vi "Scope_5782_Dual_PID.vi"() -> ()   [LabVIEW 2013]
uses:
  <vilib>/userdefined/High Color/nirio_resource_hc.ctl
  FPGA/DataMode.ctl
  <vilib>/Analysis/4window.llb/windowTd.ctl
  Host/Scope/controls/power_spectrum_unit.ctl
  Host/Scope5782/Scope/controls/5782_trigger_type.ctl
  Host/Scope/controls/Data_calc_mode.ctl
  Host/Scope/controls/Data_display_mode.ctl
  Host/Scope/controls/Graph_references.ctl
  Host/Scope/controls/graph_controls.ctl
  Host/Scope/controls/Channel_select.ctl
  Host/Communication/response.ctl
  Host/Communication/driver_status.ctl
  Host/Communication/Driver/RemoteConnection/RemoteReferences.ctl
  Host/Communication/Driver/TcpServerDriver/TcpServerDriver.lvclass
  Host/Scope5782/Scope/controls/c_t_type.ctl
  Host/Scope/controls/ScopeMode.ctl
  FPGA/fpga_settings.ctl
  Host/Communication/global_stop.vi
  <vilib>/FPGAPlugInAG/PXIe-7975R/niLvFpga_Open_PXIe-7975R.vi
  <vilib>/rvi/interface/common/dynamic/niFpgaDynamicAddResources.vi
  <vilib>/rvi/interface/common/niFpgaWaitOnOcc.vi
  <vilib>/Utility/error.llb/Error Cluster From Error Code.vi
  <vilib>/rvi/errors/niLvFpgaAdjustHostInterfaceError.vi
  <vilib>/FPGAPlugInAG/Dynamic/niLvFpga_Close_Dynamic.vi
  <vilib>/rvi/interface/nirviOpenFPGA/nirviOpenFPGA.xnode
  FPGA Bitfiles/FPGAmain_5782_Dual_PID_1Hh0+AVfYHk.lvbitx
  <vilib>/rvi/interface/nirviReadWriteControl/nirviReadWriteControl.xnode
  Host/Scope5782/Config/FPGAref_5782.ctl
  <vilib>/rvi/FXPMathLib/FxpInterpret/XNode/nifxpmath_Interpret.xnode
  <vilib>/rvi/interface/nirviMethod/nirviMethod.xnode
  <vilib>/rvi/interface/nirviCloseFPGA/nirviCloseFPGA.xnode
  Host/Utilities/Ticker/Ticker.lvclass
  NiFpgaLv.dll
  <vilib>/rvi/interface/Simulation/niFpgaSimulationCallBeginRW.vi
  Host/Communication/Driver/RemoteConnection/RemoteConnection.lvclass
  <vilib>/FPGAPlugInAG/Dynamic/niLvFpga_WriteFifo_Dynamic.vi
  <vilib>/rvi/errors/niLvFpgaMergeErrorWithErrorCode.vi
  <vilib>/Analysis/NI_AALPro.lvlib
panel:
  in  "Output enabled":bool=TRUE
  in  "unwrap phase":bool
  in  "Kp AM":fxp<+/-,32,4> caption="Kp"
  in  "Kd/T AM":fxp<+/-,32,4> caption="Kd/T"
  in  "Ki*T AM":fxp<+/-,32,4> caption="Ki*T"
  in  "Feedback AM":bool caption="Feedback"
  in  "c(t) AM":bool
  in  "c(t) phase":bool
  in  "Kp":fxp<+/-,32,4>
  in  "Kd/T":fxp<+/-,32,4>
  in  "Ki*T":fxp<+/-,32,4>
  in  "Feedback":bool
  in  "b":fxp<+/-,16,2>
  in  "a":fxp<+/-,16,2>
  in  "Fequency [kHz]":dbl format="%#_8g"
  in  "#bins":i32=1 min=1 max=16
  in  "ch1 DC offset":dbl caption="DC offset\nChannel 1"
  in  "ch0 DC offset":dbl caption="DC offset\nChannel 0"
  in  "Output delay delta":dbl(slide) scale=0.0..6.0
  in  "Output delay":dbl(slide) scale=0.0..6.0
  in  "Chart length":i32=200000
  in  "Trigmode":enum32{"Triggered", "Continuous"}(radio)
  in  "Refence for phase":T1
  in  "Graph_refs":T2
  out "Lower chart":dbl[][](graph)
  out "Upper chart":dbl[][](graph)
  out "Lower graph":i16[][](graph)
  in  "Buffer":T4
  in  "Display":T5
  in  "Output mixer fequency [MHz]":dbl
  in  "Trigger":T6
  in  "Ch1 Q":bool
  in  "Ch1 I":bool
  in  "Ch0 Q":bool
  in  "Ch0 I":bool
  in  "Ch1":bool
  in  "Ch0":bool
  out "stop 2":bool
  in  "Zoom freq X":bool
  in  "Zoom freq Y":bool
  in  "Zoom time Y":bool
  in  "Zoom time X":bool
  in  "Unit":T7
  in  "Window":T8=1 items=["Rectangle"=0, "Hanning"=1, "Hamming"=2, "Blackman-Harris"=3, "Exact Blackman"=4, "Blackman"=5, "Flat Top"=6, "4 Term B-Harris "=7, "7 Term B-Harris"=8, "Low Sidelobe"=9, "Blackman Nuttall"=11, "Triangle"=30, "Bartlett-Hanning"=31, "Bohman"=32, "Parzen"=33, "Welch"=34, "Kaiser"=60, "Dolph-Chebyshev"=61, "Gaussian"=62]
  in  "Samples per 5782 record":i32
  in  "Phase offset (deg)":dbl
  in  "Fequency [MHz]":dbl format="%#_8g"
  in  "Mode":T9
  in  "Mixer freq [MHz]":dbl
  out "freqdata":cluster{"f0":dbl, "df":dbl, "magnitude":dbl[]}[](graph)
  out "Upper graph":i16[][](graph)
  in  "Rumode":bool
  in  "Singleshot":bool
  out "error IO":errorcluster
  in  "stop":bool
  in  "resource name":T10="RIO0"
  out "Clocking Option Configured?":bool
  out "Configured?":bool
  # "FPGA setup"
  # "V"
  # "V"
  # "Output delay"
  # "ns"
  # "Auto Zoom"
  # "Output delay delta"
  # "ps"
  # "Amplitude modulation"
  # "5782"
  # "Phase"
  # "Amplitude"
  # "Simulated data"
  # "FFT"
  # "Auto Zoom"
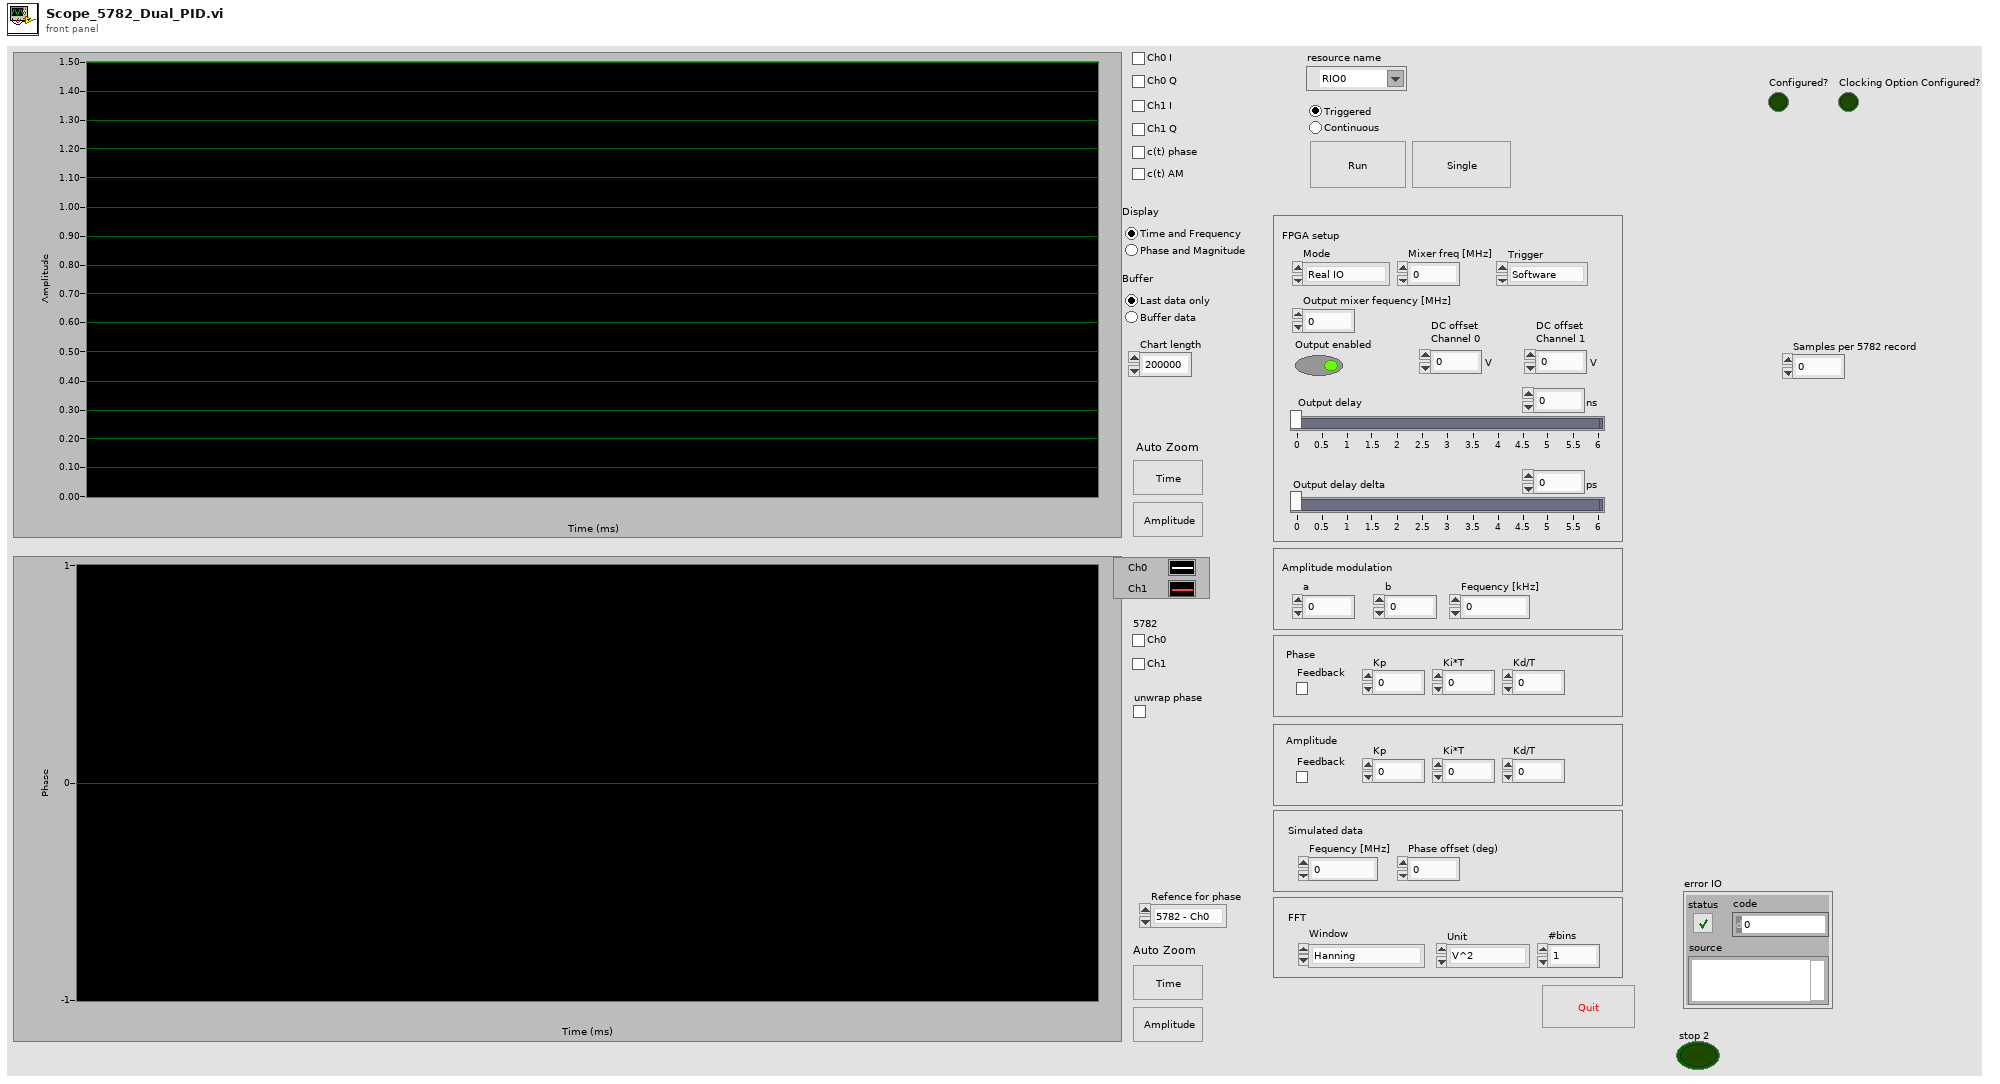
[diagram p1: front panel]
types:
  T1 = typedef "Channel_select.ctl" = enum16{"5782 - Ch0", "5782 - Ch1"}
  T2 = typedef "Graph_references.ctl" = cluster{"upper":T3, "lower":T3, "Freq graph":refnum<vi>}
  T3 = typedef "graph_controls.ctl" = cluster{"Graph":refnum<vi>, "Time btn":refnum<vi>, "Amplitude btn":refnum<vi>, "Chart":refnum<vi>}
  T4 = typedef "Data_display_mode.ctl" = enum32{"Last data only", "Buffer data"}
  T5 = typedef "Data_calc_mode.ctl" = enum32{"Time and Frequency", "Phase and Magnitude"}
  T6 = typedef "5782_trigger_type.ctl" = enum16{"Software", "Trigger input"}
  T7 = typedef "power_spectrum_unit.ctl" = enum16{"V^2", "V", "dBV"}
  T8 = typedef "NI_AALPro.lvlib/windowTd.ctl" = u32
  T9 = typedef "DataMode.ctl" = enum16{"Real IO", "Simulated"}
  T10 = typedef "nirio_resource_hc.ctl" = tag
  T11 = typedef "RemoteConnection.lvclass/RemoteReferences.ctl" = cluster{"a":refnum<vi>, "b":refnum<vi>, "fm":refnum<vi>, "Output delay":refnum<vi>, "Output delay delta":refnum<vi>}
  T12 = typedef "response.ctl" = cluster{"driver status":T13, "Sender":string, "Type":i32, "Variant":variant}
  T13 = typedef "driver_status.ctl" = enum16{"Normal", "Startup", "Connection lost", "Reconnected", "Timeout", "Idle", "Busy"}
  T14 = enum8{"Internal Clock PLL Off", "Internal Clock PLL On (REF IN)", "External Clock (CLK_IN)", "Internal Clock PLL On (IoModSyncClk)"}
  T15 = typedef "message_queue.ctl" = refnum<queue>
  T16 = typedef "FPGAref_5782.ctl" = refnum<k20>
  T17 = typedef "scope_params_5782.ctl" = cluster{"scope mode":T18, "ticker":refnum<class "Ticker.lvclass">, "samples per record":i32, "FPGA ref":T16, "data mode":T9, "5782 Trigger":T6, "Chart length":i32, "RemoteConnection":refnum<class "RemoteConnection.lvclass">, "last phase":dbl[]}
  T18 = typedef "ScopeMode.ctl" = enum16{"Stopped", "Single", "Running", "Continuous"}
  T19 = typedef "c_t_type.ctl" = enum16{"Phase", "AM", "Both"}
  T20 = typedef "fpga_settings.ctl" = enum16{"Feedback Enable", "New FIR coeffs", "FIR shift", "Enable filter", "Set Downsample", "Downsample", "CIC Gain", "Record length", "Trigger samples", "Quiet time", "a_am", "b_am", "Use fixed delay", "fixed sin_fi", "fixed cos_fi", "Ki*Tau", "Kp", "Kd_Tau", "Fi_start", "Fi_delta", "DC_offs 0", "DC_offs 1", "Ki*Tau am", "Kp am", "Kd_Tau am", "Feedback AM"}
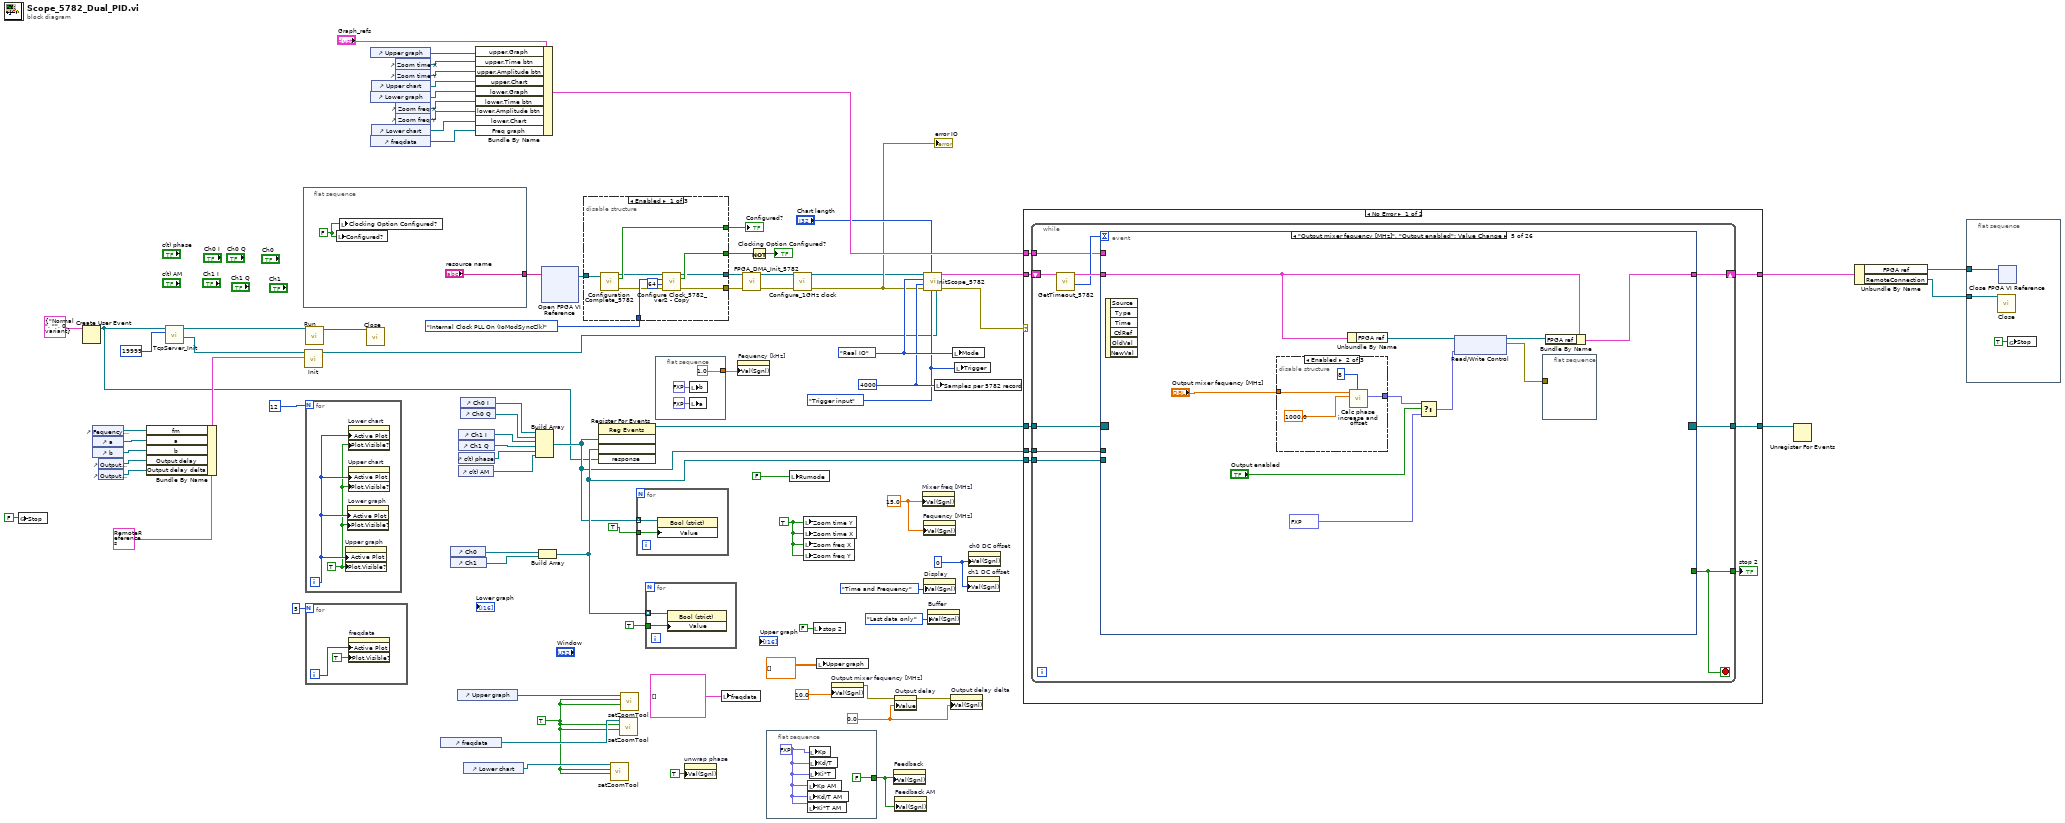
[diagram p0: block diagram]
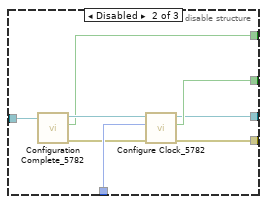
[diagram p2: hidden frame]
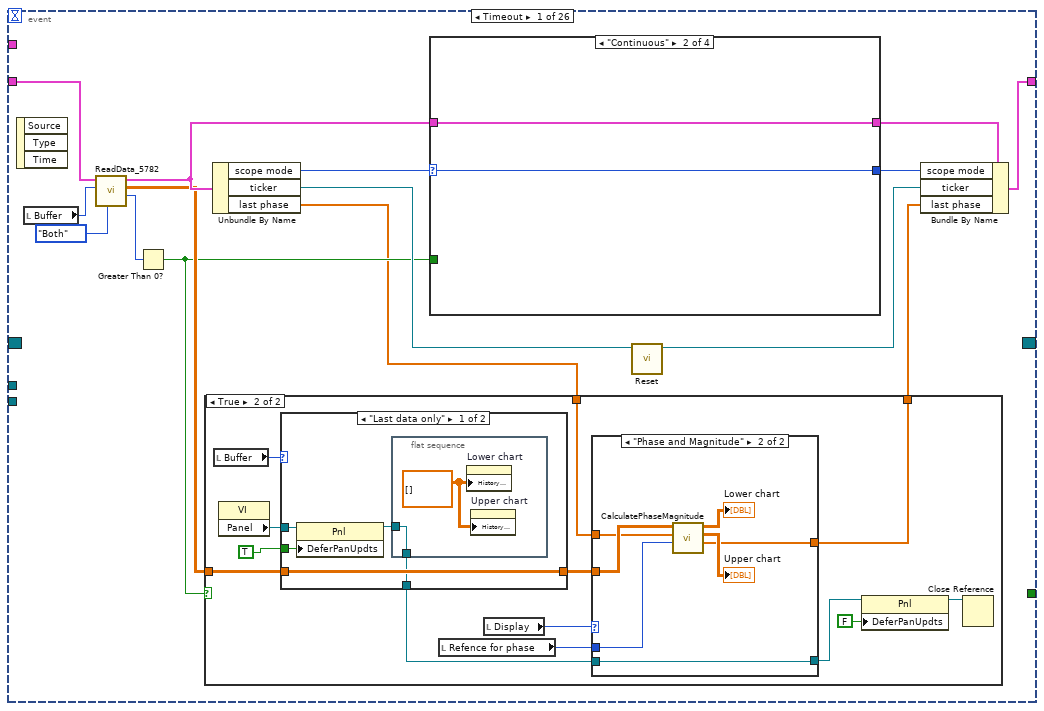
[diagram p4: hidden frame]
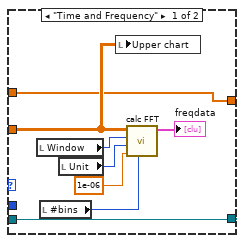
[diagram p7: hidden frame]
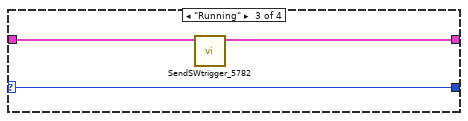
[diagram p9: hidden frame]
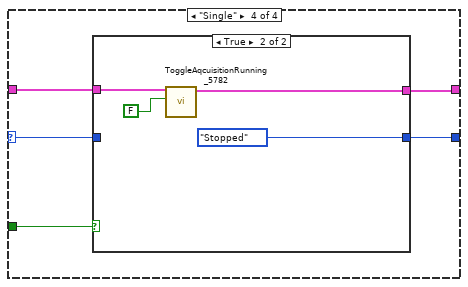
[diagram p10: hidden frame]
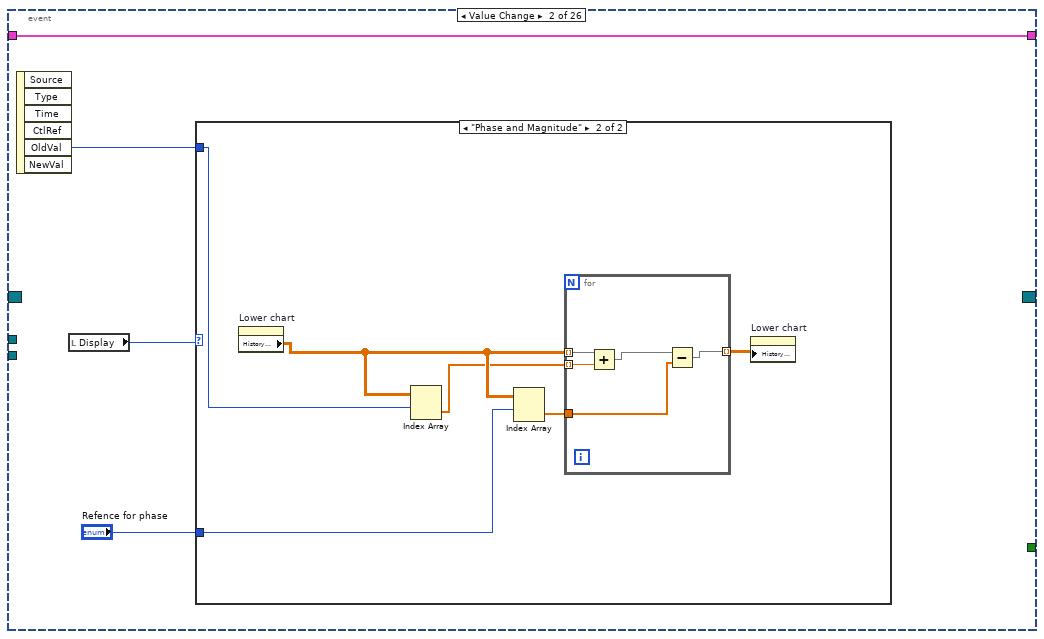
[diagram p12: hidden frame]
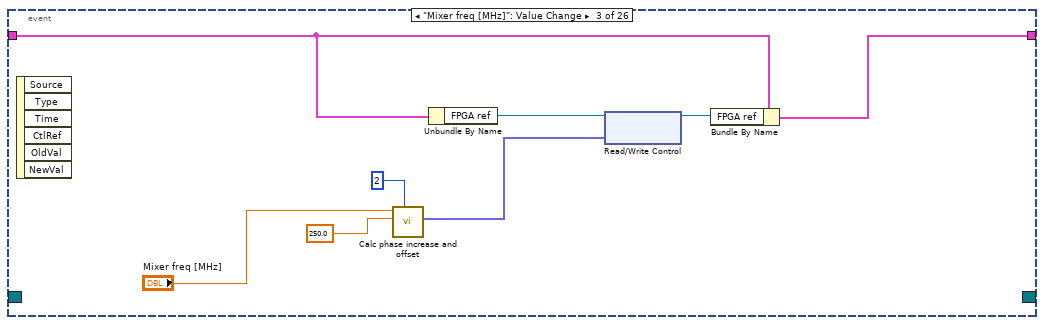
[diagram p14: hidden frame]
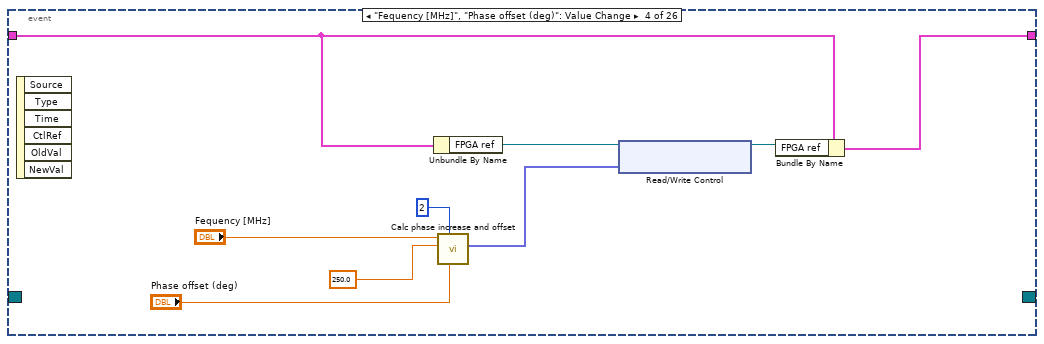
[diagram p15: hidden frame]
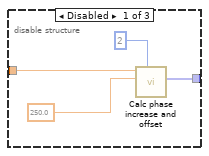
[diagram p16: hidden frame]
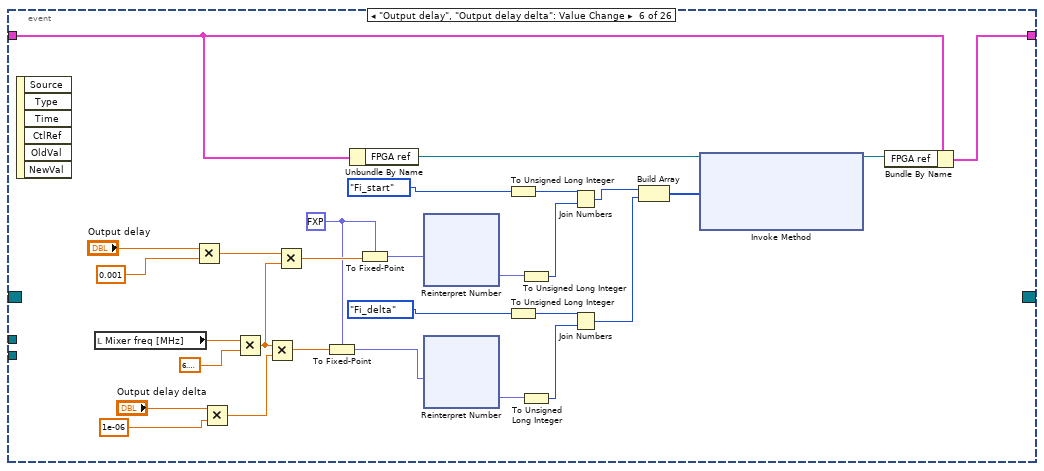
[diagram p18: hidden frame]
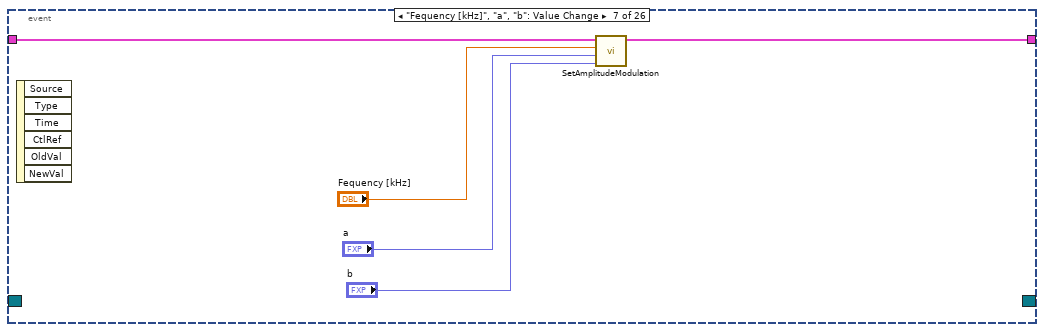
[diagram p19: hidden frame]
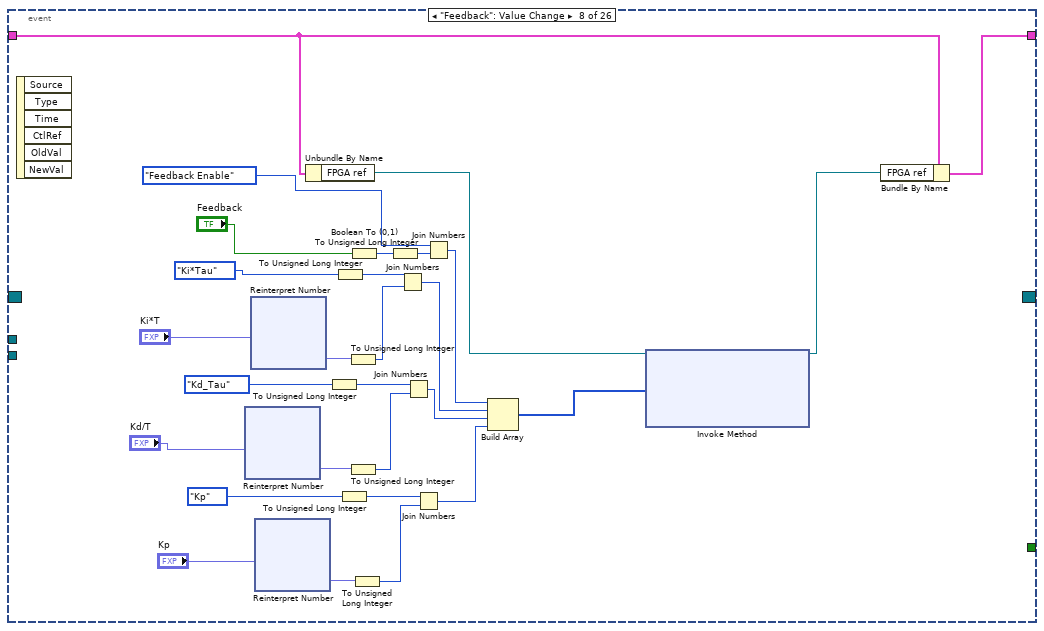
[diagram p20: hidden frame]
diagram:
  w30 = i16 0 ("Value (Signaling)")
  w31 = 0.0 ("Value (Signaling)")
  w54 = 5782_trigger_type."Trigger input" ("Trigger")
  w12 = TRUE ("Zoom  X")
  w68 = TRUE ("Rumode")
  w67 = DataMode."Real IO" ("Mode")
  w56 = 4000 ("Samples to aqcuire")
  w79 = 15.0 ("Mixer requency [MHz]")
  n1 = global write "global_stop.vi" "Stop"(FALSE ("Stop")) -> ()
  n2 = Create User Event(user event datatype=T12 {"driver status"=enum."Normal", "Sender"="", "Type"=0, "Variant"=variant} ("response")) -> (user event=w18:refnum<user-event>)  [unwired: 1 in, 1 out]
  n3 = control-ref of="Fequency [kHz]"() -> (w20:refnum<vi>)
  n4 = control-ref of="a"() -> (w21:refnum<vi>)
  n5 = control-ref of="b"() -> (w19:refnum<vi>)
  n6 = control-ref of="Output delay"() -> (w3:refnum<vi>)
  n7 = control-ref of="Output delay delta"() -> (w2:refnum<vi>)
  n8 = Bundle By Name(cluster=T11 {"a"=refnum, "b"=refnum, "fm"=refnum, "Output delay"=refnum, "Output delay delta"=refnum} ("refs"), "fm"=w20, "a"=w21, "b"=w19, "Output delay"=w3, "Output delay delta"=w2) -> (w28:T11)
  n9 = call "TcpServer_Init.vi"("local port"=u16 19999, "response event"=w18) -> ("Message queue"=w26:T15, "TcpServerDriver"=w23:refnum<class "TcpServerDriver.lvclass">)  [unwired: 8 in]
  n10 = flat-sequence {
    tunnel: ["resource name"] -> w69
    frame #0 {
      w84 = FALSE ("Trigger Acquisition")
      n11 = local write "Configured?"(w84) -> ()
      n12 = local write "Clocking Option Configured?"(w84) -> ()
    }
  }
  n13 = call "Init.vi"("refs"=w28, "server queue"=w26) -> ("RemoteConnection"=w17:refnum<class "RemoteConnection.lvclass">)  [unwired: 9 in]
  n14 = for {
    N: 12 -> [_]
    i -> [w87]
    w86 = TRUE ("Plot.Visible")
    n15 = property on="Upper graph" class="WFGraph (strict)"("Active Plot"=w87, "Plot.Visible?"=w86) -> ()  [unwired: 2 in, 2 out]
    n16 = property on="Lower graph" class="WFGraph (strict)"("Active Plot"=w87, "Plot.Visible?"=w86) -> ()  [unwired: 2 in, 2 out]
    n17 = property on="Lower chart" class="WFChart (strict)"("Active Plot"=w87, "Plot.Visible?"=w86) -> ()  [unwired: 2 in, 2 out]
    n18 = property on="Upper chart" class="WFChart (strict)"("Active Plot"=w87, "Plot.Visible?"=w86) -> ()  [unwired: 2 in, 2 out]
  }
  n19 = for {
    N: 5 -> [_]
    i -> [w88]
    n20 = property on="freqdata" class="WFGraph (strict)"("Active Plot"=w88, "Plot.Visible?"=TRUE ("Plot.Visible")) -> ()  [unwired: 2 in, 2 out]
  }
  n21 = call-dynamic "Run.vi"("BaseDriver in"=w23) -> ("BaseDriver out"=w24:refnum<class "TcpServerDriver.lvclass">)  [unwired: 9 in, 1 out]
  n22 = call-dynamic "Close.vi"("BaseDriver in"=w24) -> ()  [unwired: 9 in, 2 out]
  n23 = control-ref of="Upper graph"() -> (w51:refnum<vi>)
  n24 = control-ref of="Lower graph"() -> (w47:refnum<vi>)
  n25 = control-ref of="freqdata"() -> (w43:refnum<vi>)
  n26 = control-ref of="Upper chart"() -> (w48:refnum<vi>)
  n27 = control-ref of="Lower chart"() -> (w44:refnum<vi>)
  n28 = control-ref of="Zoom time X"() -> (w50:refnum<vi>)
  n29 = control-ref of="Zoom time Y"() -> (w49:refnum<vi>)
  n30 = control-ref of="Zoom freq X"() -> (w46:refnum<vi>)
  n31 = control-ref of="Zoom freq Y"() -> (w45:refnum<vi>)
  n32 = control-ref of="freqdata"() -> (w57:refnum<vi>)
  n33 = control-ref of="Ch0"() -> (w64:refnum<vi>)
  n34 = control-ref of="Ch1"() -> (w65:refnum<vi>)
  n35 = control-ref of="Upper graph"() -> (w58:refnum<vi>)
  n36 = control-ref of="c(t) AM"() -> (w5:refnum<vi>)
  n37 = control-ref of="Ch1 I"() -> (w62:refnum<vi>)
  n38 = control-ref of="Ch1 Q"() -> (w63:refnum<vi>)
  n39 = control-ref of="c(t) phase"() -> (w6:refnum<vi>)
  n40 = control-ref of="Ch0 I"() -> (w60:refnum<vi>)
  n41 = control-ref of="Ch0 Q"() -> (w61:refnum<vi>)
  n42 = control-ref of="Lower chart"() -> (w13:refnum<vi>)
  n43 = Bundle By Name(cluster="Graph_refs", "upper.Graph"=w51, "upper.Time btn"=w50, "upper.Amplitude btn"=w49, "upper.Chart"=w48, "lower.Graph"=w47, "lower.Time btn"=w46, "lower.Amplitude btn"=w45, "lower.Chart"=w44, "Freq graph"=w43) -> (w42:T2)
  n44 = Build Array(w60, w61, w62, w63, w6, w5) -> (w59:refnum<vi>[])
  n45 = Build Array(w64, w65) -> (w71:refnum<vi>[])
  n46 = xnode "Open FPGA VI Reference"("resource name"=w69) -> ("FPGA VI Reference Out"=w36:refnum<k20>)  [unwired: 1 in, 1 out]
  n47 = disable-structure shown="Enabled" {
    disable-tunnel: [w98 w106 _] -> w38
    disable-tunnel: T14."Internal Clock PLL On (IoModSyncClk)" ("Clock Source") -> [w97 w105 _]
    disable-tunnel: [w95 w103 _] -> w37
    disable-tunnel: [w94 w100 w107] -> w11
    disable-tunnel: w36 -> [w92 w102 w107]
    disable-tunnel: [w93 w99 _] -> w34
    frame Enabled {
      n48 = call "Configuration Complete_5782.vi"("FPGA VI Reference in"=w92) -> ("error out"=w96:errorcluster, "Configured?"=w93:bool, "FPGA VI Reference out"=w91:refnum<k20>)  [unwired: 8 in]
      n49 = call "Configure Clock_5782_ver2 - Copy.vi"("error in"=w96, "User Data 1"=u8 64, "Clock Source"=w97, "FPGA VI Reference"=w91) -> ("error out"=w95:errorcluster, "Configuration Error"=w98:bool, "FPGA VI Reference out"=w94:refnum<k20>)  [unwired: 5 in]
    }
    frame Disabled {
      n50 = call "Configuration Complete_5782.vi"("FPGA VI Reference in"=w102) -> ("error out"=w104:errorcluster, "Configured?"=w99:bool, "FPGA VI Reference out"=w101:refnum<k20>)  [unwired: 8 in]
      n51 = call "Configure Clock_5782.vi"("error in"=w104, "Clock Source"=w105, "FPGA VI Reference in"=w101) -> ("error out"=w103:errorcluster, "Configuration Error"=w106:bool, "FPGA VI Reference Out"=w100:T16)  [unwired: 6 in]
    }
    frame Disabled {
    }
  }
  "Configured?" <- w34
  n52 = register-events(w59, w71, w18) -> (reference out=w75:refnum<event-registration>)  [unwired: 2 in, 1 out]
  n53 = call "setZoomTool.vi"("Zoom Y"=w12, "Zoom  X"=w12, "reference"=w13) -> ()  [unwired: 9 in]
  n54 = call "setZoomTool.vi"("Zoom Y"=w12, "Zoom  X"=w12, "reference"=w57) -> ()  [unwired: 9 in]
  n55 = call "setZoomTool.vi"("Zoom Y"=w12, "Zoom  X"=w12, "reference"=w58) -> ()  [unwired: 9 in]
  n56 = for {
    tunnel: w59 -> [w109] mode=indexing
    tunnel: TRUE ("Rumode") -> [w108]
    n57 = property class="Bool (strict)"(reference=w109, "Value"=w108) -> ()  [unwired: 1 in, 2 out]
  }
  n58 = for {
    tunnel: w71 -> [w111] mode=indexing
    tunnel: TRUE ("Rumode") -> [w110]
    n59 = property class="Bool (strict)"(reference=w111, "Value"=w110) -> ()  [unwired: 1 in, 2 out]
  }
  n60 = flat-sequence {
    tunnel: [1.0 ("Value (Signaling)")] -> w29
    frame #0 {
      n61 = local write "b"(fxp<+/-,16,2> 0.0 ("b")) -> ()
      n62 = local write "a"(fxp<+/-,16,2> 1.0 ("a")) -> ()
    }
  }
  n63 = property on="unwrap phase" class="Bool (strict)"("Val(Sgnl)"=TRUE ("Value (Signaling)")) -> ()  [unwired: 2 in, 2 out]
  n64 = local write "freqdata"(cluster{"f0":dbl, "df":dbl, "magnitude":dbl[]}[] [] ("freqdata")) -> ()
  n65 = property on="Fequency [kHz]" class="DigNum (strict)"("Val(Sgnl)"=w29) -> ()  [unwired: 2 in, 2 out]
  n66 = call "FPGA_DMA_Init_5782.vi"("error in (no error)"=w37, "FPGA VI Reference"=w11) -> ("error out"=w9:errorcluster, "FPGA VI Out"=w10:refnum<k20>)  [unwired: 7 in, 1 out]
  n67 = Not(x=w38) -> (.not. x?=→"Clocking Option Configured?":bool)
  n68 = flat-sequence {
    tunnel: [FALSE] -> w4
    frame #0 {
      w115 = fxp<+/-,32,4> 0.0 ("Kp")
      n69 = local write "Kp AM"(w115) -> ()
      n70 = local write "Kd/T AM"(w115) -> ()
      n71 = local write "Ki*T AM"(w115) -> ()
      n72 = local write "Kp"(w115) -> ()
      n73 = local write "Kd/T"(w115) -> ()
      n74 = local write "Ki*T"(w115) -> ()
    }
  }
  n75 = local write "Rumode"(FALSE ("Rumode")) -> ()
  n76 = call "Configure_1GHz clock.vi"("error in"=w9, "FPGA SPI config ref"=w10) -> ("error out"=w8:errorcluster, "FPGA SPI config out"=w7:refnum<k20>)  [unwired: 8 in]
  "error IO" <- w8
  n77 = local write "Zoom time Y"(w68) -> ()
  n78 = local write "Zoom time X"(w68) -> ()
  n79 = local write "Zoom freq X"(w68) -> ()
  n80 = local write "Zoom freq Y"(w68) -> ()
  n81 = local write "stop 2"(FALSE ("stop 2")) -> ()
  n82 = local write "Upper graph"(dbl[][] [] ("Timedata")) -> ()
  n83 = property on="Output mixer fequency [MHz]" class="DigNum (strict)"("Val(Sgnl)"=10.0 ("Mixer requency [MHz]")) -> (error out=w32:errorcluster)  [unwired: 2 in, 1 out]
  n84 = property on="Feedback" class="Bool (strict)"("Val(Sgnl)"=w4) -> ()  [unwired: 2 in, 2 out]
  n85 = property on="Output delay" class="Slide (strict)"(error in=w32, "Value"=w31) -> (error out=w33:errorcluster)  [unwired: 1 in, 1 out]
  n86 = property on="Feedback AM" class="Bool (strict)"("Val(Sgnl)"=w4) -> ()  [unwired: 2 in, 2 out]
  n87 = property on="Mixer freq [MHz]" class="DigNum (strict)"("Val(Sgnl)"=w79) -> ()  [unwired: 2 in, 2 out]
  n88 = property on="Fequency [MHz]" class="DigNum (strict)"("Val(Sgnl)"=w79) -> ()  [unwired: 2 in, 2 out]
  n89 = call "InitScope_5782.vi"("RemoteConnection"=w17, "Trigger"=w54, "Chart length"="Chart length", "error in"=w8, "Samples Per Trigger"=w56, "data mode"=w67, "FPGA ref"=w7) -> ("error out"=w14:errorcluster, "scope params"=w83:T17)  [unwired: 3 in]
  n90 = property on="Display" class="RadioBtnsControl (strict)"("Val(Sgnl)"=Data_calc_mode."Time and Frequency" ("Value (Signaling)")) -> ()  [unwired: 2 in, 2 out]
  n91 = property on="Buffer" class="RadioBtnsControl (strict)"("Val(Sgnl)"=enum32{"Last data only", "Buffer data"}."Last data only" ("Value (Signaling)")) -> ()  [unwired: 2 in, 2 out]
  n92 = local write "Samples per 5782 record"(w56) -> ()
  n93 = property on="Output delay delta" class="Slide (strict)"(error in=w33, "Val(Sgnl)"=w31) -> ()  [unwired: 1 in, 2 out]
  n94 = local write "Mode"(w67) -> ()
  n95 = local write "Trigger"(w54) -> ()
  n96 = property on="ch1 DC offset" class="DigNum (strict)"("Val(Sgnl)"=w30) -> ()  [unwired: 2 in, 2 out]
  n97 = property on="ch0 DC offset" class="DigNum (strict)"("Val(Sgnl)"=w30) -> ()  [unwired: 2 in, 2 out]
  n98 = case shown="No Error" w14 {
    tunnel: w83 -> [w124 w496]
    tunnel: [w123 w496] -> w55
    tunnel: w75 -> [w122 w495]
    tunnel: [w121 w495] -> w74
    tunnel: w59 -> [w120 _]
    tunnel: w71 -> [w119 _]
    tunnel: w42 -> [w117 _]
    frame No Error {
      n99 = while {
        shift-right: [w134] -> w123
        shift-left: w124 -> [w133]
        tunnel: w122 -> [w130]
        tunnel: [w129] -> w121
        tunnel: w120 -> [w128]
        tunnel: w119 -> [w127]
        tunnel: [w126] -> w118
        tunnel: w117 -> [w125]
        stop <- w126 stop-if-true
        n100 = call "GetTimeout_5782.vi"("scope in"=w133) -> ("Time left"=w131:i32, "scope out"=w132:T17)  [unwired: 9 in]
        n101 = event shown="[4] \"Output mixer fequency [MHz]\", \"Output enabled\": Value Change" {
          selector: w130 -> [_ _ _ _ _ _ _ _ _ _ _ _ _ _ _ _ _ _ _ _ _ _ _ _ _ _]
          dyn-events: [_ _ _ _ _ _ _ _ _ _ _ _ _ _ _ _ _ _ _ _ _ _ _ _ _ _] -> w129
          timeout: w131 -> [_ _ _ _ _ _ _ _ _ _ _ _ _ _ _ _ _ _ _ _ _ _ _ _ _ _]
          tunnel: [_ _ _ _ _ _ _ _ _ _ _ _ _ _ _ _ _ _ _ _ "stop" _ _ _ _ _] -> w126
          tunnel: w132 -> [w144 w209 w227 w233 w247 w282 w289 w317 w345 w359 w373 w377 w381 w384 w394 w402 w427 w438 w451 w456 w459 w466 w476 w481 w487 w494]
          tunnel: [w147 w209 w225 w232 w246 w281 w288 w316 w344 w358 w372 w376 w380 w383 w391 w399 w427 w438 w451 w455 w459 w466 w476 w481 w487 w494] -> w134
          tunnel: w128 -> [_ _ _ _ _ _ _ _ _ _ _ _ _ _ _ _ w426 _ _ _ _ _ _ _ _ _]
          tunnel: w127 -> [_ _ _ _ _ _ _ _ _ _ _ _ _ _ _ _ _ w436 _ _ _ _ _ _ _ _]
          tunnel: w125 -> [_ _ _ _ _ _ _ _ _ _ _ _ _ _ _ _ _ _ _ _ _ _ _ _ _ w491]
          event Timeout {
            n102 = event-data() -> ()  [unwired: 1 in, 3 out]
            n103 = local read "Buffer"() -> (w138:T4)
            n104 = call "ReadData_5782.vi"("c(t)"=c_t_type."Both", "Buffer mode"=w138, "scope params"=w144) -> ("Num elements"=w140:i32, "data"=w141:dbl[][], "scope params out"=w143:T17)  [unwired: 6 in]
            n105 = Greater Than 0?(x=w140) -> (x > 0?=w139:bool)
            n106 = Unbundle By Name(w143) -> ("scope mode"=w146:T18, "ticker"=w149:refnum<class "Ticker.lvclass">, "last phase"=w137:dbl[])
            n107 = case shown="True" w139 {
              tunnel: w141 -> [_ w160]
              tunnel: w137 -> [w150 w152]
              tunnel: [w150 w151] -> w136
              frame False {
              }
              frame True {
                n108 = local read "Buffer"() -> (w162:T4)
                n109 = property class="VI"() -> ("Panel"=w155:refnum<vi>)  [unwired: 2 in, 2 out]
                n110 = case shown="\"Last data only\"" w162 {
                  tunnel: w160 -> [w168 w172]
                  tunnel: [w168 w172] -> w161
                  tunnel: w155 -> [w167 w171]
                  tunnel: TRUE ("Defer Panel Updates") -> [w165 _]
                  tunnel: [w164 w171] -> w153
                  frame "Last data only" {
                    n111 = property class="Pnl"(reference=w167, "DeferPanUpdts"=w165) -> (reference out=w166:refnum<vi>)  [unwired: 1 in, 1 out]
                    n112 = flat-sequence {
                      tunnel: w166 -> [w169]
                      tunnel: [w169] -> w164
                      frame #0 {
                        w170 = dbl[][] [] ("History Data")
                        n113 = property on="Lower chart" class="WFChart (strict)"("History Data"=w170) -> ()  [unwired: 2 in, 2 out]
                        n114 = property on="Upper chart" class="WFChart (strict)"("History Data"=w170) -> ()  [unwired: 2 in, 2 out]
                      }
                    }
                  }
                  frame "Buffer data" {
                  }
                }
                n115 = local read "Refence for phase"() -> (w159:T1)
                n116 = local read "Display"() -> (w163:T5)
                n117 = case shown="\"Phase and Magnitude\"" w163 {
                  tunnel: w161 -> [w176 w187]
                  tunnel: w159 -> [_ w184]
                  tunnel: [w175 w183] -> w157
                  tunnel: w153 -> [w175 w183]
                  tunnel: w152 -> [w173 w182]
                  tunnel: [w173 w181] -> w151
                  frame "Time and Frequency" {
                    n118 = local read "Window"() -> (w177:T8)
                    n119 = local read "#bins"() -> (w174:i32)
                    n120 = local read "Unit"() -> (w178:T7)
                    n121 = local write "Upper chart"(w176) -> ()
                    n122 = call "calc FFT.vi"("#bins"=w174, "dt"=1e-06, "Unit"=w178, "Window"=w177, "data"=w176) -> ("Power Spectrum / PSD"=→"freqdata":cluster{"f0":dbl, "df":dbl, "magnitude":dbl[]}[])  [unwired: 6 in]
                  }
                  frame "Phase and Magnitude" {
                    n123 = call "CalculatePhaseMagnitude.vi"("phase reference channel"=w184, "previous phase"=w182, "data"=w187) -> ("last phase"=w181:dbl[], "Magnitude"=→"Upper chart":dbl[][], "Phase"=→"Lower chart":dbl[][])  [unwired: 6 in]
                  }
                }
                n124 = property class="Pnl"(reference=w157, "DeferPanUpdts"=FALSE ("Defer Panel Updates")) -> (reference out=w156:refnum<vi>)  [unwired: 1 in, 1 out]
                n125 = Close Reference(reference=w156) -> ()  [unwired: 1 in, 1 out]
              }
            }
            n126 = case shown="\"Continuous\"" w146 {
              selector: w146 -> [w189 w191 w194 w195]
              tunnel: [w189 w191 w194 w199] -> w145
              tunnel: w143 -> [w188 w190 w193 w197]
              tunnel: [w188 w190 w192 w196] -> w142
              tunnel: w139 -> [_ _ _ w198]
              frame "Stopped" {
              }
              frame "Continuous" {
              }
              frame "Running" {
                n127 = call "SendSWtrigger_5782.vi"("scope in"=w193) -> ("scope out"=w192:T17)  [unwired: 9 in, 1 out]
              }
              frame "Single" {
                n128 = case shown="True" w198 {
                  tunnel: [w200 ScopeMode."Stopped" ("scope mode")] -> w199
                  tunnel: w197 -> [w201 w204]
                  tunnel: [w201 w203] -> w196
                  tunnel: w195 -> [w200 _]
                  frame False {
                  }
                  frame True {
                    n129 = call "ToggleAqcuisitionRunning_5782.vi"("Acquisition running"=FALSE, "scope in"=w204) -> ("scope out"=w203:T17)  [unwired: 8 in, 1 out]
                  }
                }
              }
            }
            n130 = call "Reset.vi"("Ticker in"=w149) -> ("Ticker out"=w148:refnum<class "Ticker.lvclass">)  [unwired: 9 in, 1 out]
            n131 = Bundle By Name(cluster=w142, "scope mode"=w145, "ticker"=w148, "last phase"=w136) -> (w147:T17)
          }
          event Value Change {
            n132 = event-data() -> ("OldVal"=w206:T1)  [unwired: 1 in, 5 out]
            n133 = local read "Display"() -> (w207:T5)
            n134 = case shown="\"Phase and Magnitude\"" w207 {
              tunnel: "Refence for phase" -> [_ w214]
              tunnel: w206 -> [_ w212]
              frame "Time and Frequency", Default {
              }
              frame "Phase and Magnitude" {
                n135 = property on="Lower chart" class="WFChart (strict)"() -> ("History Data"=w213:dbl[][])  [unwired: 2 in, 2 out]
                n136 = Index Array(array=w213, index (row)=w212) -> (element=w211:dbl[])  [unwired: 1 in]
                n137 = Index Array(array=w213, index (row)=w214) -> (element=w215:dbl[])  [unwired: 1 in]
                n138 = for {
                  tunnel: w213 -> [w218] mode=indexing
                  tunnel: w215 -> [w220]
                  tunnel: [w219] -> w210 mode=indexing
                  tunnel: w211 -> [w217] mode=indexing
                  n139 = Add(x=w218, y=w217) -> (x+y=w216:dbl[])
                  n140 = Subtract(x=w216, y=w220) -> (x-y=w219:dbl[])
                }
                n141 = property on="Lower chart" class="WFChart (strict)"("History Data"=w210) -> ()  [unwired: 2 in, 2 out]
              }
            }
          }
          event "Mixer freq [MHz]": Value Change {
            n142 = event-data() -> ()  [unwired: 1 in, 6 out]
            n143 = call "Calc phase increase and offset.vi"("# of DDS"=2, "fclk (MHz)"=250.0 ("fclk (800MHz)"), "f_generated (MHz)"="Mixer freq [MHz]") -> ("Phase out"=w221:fxp<+,64,64>[])  [unwired: 6 in, 2 out]
            n144 = Unbundle By Name(w227) -> ("FPGA ref"=w228:T16)
            n145 = xnode "Read/Write Control"("FPGA VI Reference In"=w228, "Phase 5782"=w221) -> ("FPGA VI Reference Out"=w226:T16)  [unwired: 1 in, 1 out]
            n146 = Bundle By Name(cluster=w227, "FPGA ref"=w226) -> (w225:T17)
          }
          event "Fequency [MHz]", "Phase offset (deg)": Value Change {
            n147 = event-data() -> ()  [unwired: 1 in, 6 out]
            n148 = Unbundle By Name(w233) -> ("FPGA ref"=w235:T16)
            n149 = call "Calc phase increase and offset.vi"("Phase offset (deg)"="Phase offset (deg)", "# of DDS"=2, "fclk (MHz)"=250.0 ("fclk (800MHz)"), "f_generated (MHz)"="Fequency [MHz]") -> ("Phase out"=w229:fxp<+,64,64>[])  [unwired: 5 in, 2 out]
            n150 = xnode "Read/Write Control"("FPGA VI Reference In"=w235, "Simulated phase 5782"=w229) -> ("FPGA VI Reference Out"=w234:T16)  [unwired: 1 in, 1 out]
            n151 = Bundle By Name(cluster=w233, "FPGA ref"=w234) -> (w232:T17)
          }
          event "Output mixer fequency [MHz]", "Output enabled": Value Change {
            n152 = event-data() -> ()  [unwired: 1 in, 6 out]
            n153 = disable-structure shown="Enabled" {
              disable-tunnel: [w249 w253 _] -> w239
              disable-tunnel: "Output mixer fequency [MHz]" -> [w248 w252 _]
              frame Disabled {
                n154 = call "Calc phase increase and offset.vi"("# of DDS"=2, "fclk (MHz)"=250.0 ("fclk (800MHz)"), "f_generated (MHz)"=w248) -> ("Phase out"=w249:fxp<+,64,64>[])  [unwired: 6 in, 2 out]
              }
              frame Enabled {
                n155 = call "Calc phase increase and offset.vi"("# of DDS"=8, "fclk (MHz)"=1000.0 ("fclk (800MHz)"), "f_generated (MHz)"=w252) -> ("Phase out"=w253:fxp<+,64,64>[])  [unwired: 6 in, 2 out]
              }
              frame Disabled {
              }
            }
            n156 = Unbundle By Name(w247) -> ("FPGA ref"=w243:T16)
            n157 = Select(t=w239, s="Output enabled", f=fxp<+,64,64>[] [0.0, 0.0, 0.0, 0.0, 0.0, 0.0, 0.0, 0.0]) -> (s? t:f=w238:fxp<+,64,64>[])
            n158 = xnode "Read/Write Control"("FPGA VI Reference In"=w243, "Phase output"=w238) -> ("FPGA VI Reference Out"=w242:T16, "error out"=w244:errorcluster)  [unwired: 1 in]
            n159 = flat-sequence {
              tunnel: w244 -> [_]
              frame #0 {
              }
            }
            n160 = Bundle By Name(cluster=w247, "FPGA ref"=w242) -> (w246:T17)
          }
          event "Output delay", "Output delay delta": Value Change {
            w261 = fxp<+/-,32,4> 0.0 ("x")
            n161 = event-data() -> ()  [unwired: 1 in, 6 out]
            n162 = local read "Mixer freq [MHz]"() -> (w276:dbl)
            n163 = Multiply(x="Output delay", y=0.001) -> (x*y=w277:dbl)
            n164 = Multiply(x="Output delay delta", y=1e-06) -> (x*y=w279:dbl)
            n165 = Multiply(x=w276, y=6.283185307179586) -> (x*y=w274:dbl)
            n166 = Multiply(x=w274, y=w279) -> (x*y=w262:dbl)
            n167 = Multiply(x=w277, y=w274) -> (x*y=w264:dbl)
            n168 = To Fixed-Point(fixed-point type=w261, number=w262) -> (fixed-point=w260:fxp<+/-,32,4>)
            n169 = Unbundle By Name(w282) -> ("FPGA ref"=w257:T16)
            n170 = To Fixed-Point(fixed-point type=w261, number=w264) -> (fixed-point=w263:fxp<+/-,32,4>)
            n171 = xnode "Reinterpret Number"("x"=w263) -> ("y"=w270:fxp<+,32,32>)
            n172 = xnode "Reinterpret Number"("x"=w260) -> ("y"=w269:fxp<+,32,32>)
            n173 = To Unsigned Long Integer(number=fpga_settings."Fi_start" ("FPGA Setting")) -> (unsigned 32bit integer=w273:u32)
            n174 = To Unsigned Long Integer(number=fpga_settings."Fi_delta" ("FPGA Setting")) -> (unsigned 32bit integer=w266:u32)
            n175 = To Unsigned Long Integer(number=w270) -> (unsigned 32bit integer=w272:u32)
            n176 = To Unsigned Long Integer(number=w269) -> (unsigned 32bit integer=w267:u32)
            n177 = Join Numbers(hi=w273, lo=w272) -> ((hi.lo)=w258:u64)
            n178 = Join Numbers(hi=w266, lo=w267) -> ((hi.lo)=w259:u64)
            n179 = Build Array(w258, w259) -> (w265:u64[])
            n180 = xnode "Invoke Method"("FPGA VI Reference In"=w257, "Data"=w265) -> ("FPGA VI Reference Out"=w256:T16)  [unwired: 2 in, 2 out]
            n181 = Bundle By Name(cluster=w282, "FPGA ref"=w256) -> (w281:T17)
          }
          event "Fequency [kHz]", "a", "b": Value Change {
            n182 = event-data() -> ()  [unwired: 1 in, 6 out]
            n183 = call "SetAmplitudeModulation.vi"("b_am"="b", "a_am"="a", "Am freq [kHz]"="Fequency [kHz]", "scope in"=w289) -> ("scope out"=w288:T17)  [unwired: 7 in]
          }
          event "Feedback": Value Change {
            n184 = event-data() -> ()  [unwired: 1 in, 6 out]
            n185 = xnode "Reinterpret Number"("x"="Kd/T") -> ("y"=w303:fxp<+,32,32>)
            n186 = xnode "Reinterpret Number"("x"="Ki*T") -> ("y"=w300:fxp<+,32,32>)
            n187 = xnode "Reinterpret Number"("x"="Kp") -> ("y"=w307:fxp<+,32,32>)
            n188 = Unbundle By Name(w317) -> ("FPGA ref"=w315:T16)
            n189 = To Unsigned Long Integer(number=fpga_settings."Kd_Tau" ("FPGA Setting")) -> (unsigned 32bit integer=w301:u32)
            n190 = To Unsigned Long Integer(number=fpga_settings."Ki*Tau" ("FPGA Setting")) -> (unsigned 32bit integer=w297:u32)
            n191 = To Unsigned Long Integer(number=fpga_settings."Kp" ("FPGA Setting")) -> (unsigned 32bit integer=w304:u32)
            n192 = To Unsigned Long Integer(number=w300) -> (unsigned 32bit integer=w296:u32)
            n193 = To Unsigned Long Integer(number=w303) -> (unsigned 32bit integer=w302:u32)
            n194 = Boolean To (0,1)(Boolean="Feedback") -> (0, 1=w312:i16)
            n195 = To Unsigned Long Integer(number=w307) -> (unsigned 32bit integer=w306:u32)
            n196 = To Unsigned Long Integer(number=w312) -> (unsigned 32bit integer=w309:u32)
            n197 = Join Numbers(hi=w297, lo=w296) -> ((hi.lo)=w295:u64)
            n198 = Join Numbers(hi=w301, lo=w302) -> ((hi.lo)=w294:u64)
            n199 = Join Numbers(hi=w304, lo=w306) -> ((hi.lo)=w314:u64)
            n200 = Join Numbers(hi=fpga_settings."Feedback Enable" ("FPGA Setting"), lo=w309) -> ((hi.lo)=w310:u64)
            n201 = Build Array(w310, w295, w294, w314) -> (w313:u64[])
            n202 = xnode "Invoke Method"("FPGA VI Reference In"=w315, "Data"=w313) -> ("FPGA VI Reference Out"=w290:T16)  [unwired: 2 in, 2 out]
            n203 = Bundle By Name(cluster=w317, "FPGA ref"=w290) -> (w316:T17)
          }
          event "Feedback AM": Value Change {
            n204 = event-data() -> ()  [unwired: 1 in, 6 out]
            n205 = xnode "Reinterpret Number"("x"="Kd/T AM") -> ("y"=w332:fxp<+,32,32>)
            n206 = xnode "Reinterpret Number"("x"="Ki*T AM") -> ("y"=w329:fxp<+,32,32>)
            n207 = xnode "Reinterpret Number"("x"="Kp AM") -> ("y"=w336:fxp<+,32,32>)
            n208 = Unbundle By Name(w345) -> ("FPGA ref"=w343:T16)
            n209 = To Unsigned Long Integer(number=fpga_settings."Kd_Tau am" ("FPGA Setting")) -> (unsigned 32bit integer=w330:u32)
            n210 = To Unsigned Long Integer(number=fpga_settings."Ki*Tau am" ("FPGA Setting")) -> (unsigned 32bit integer=w328:u32)
            n211 = To Unsigned Long Integer(number=fpga_settings."Kp am" ("FPGA Setting")) -> (unsigned 32bit integer=w333:u32)
            n212 = To Unsigned Long Integer(number=w329) -> (unsigned 32bit integer=w327:u32)
            n213 = To Unsigned Long Integer(number=w332) -> (unsigned 32bit integer=w331:u32)
            n214 = Boolean To (0,1)(Boolean="Feedback AM") -> (0, 1=w340:i16)
            n215 = To Unsigned Long Integer(number=w336) -> (unsigned 32bit integer=w335:u32)
            n216 = To Unsigned Long Integer(number=w340) -> (unsigned 32bit integer=w337:u32)
            n217 = Join Numbers(hi=w328, lo=w327) -> ((hi.lo)=w326:u64)
            n218 = Join Numbers(hi=w330, lo=w331) -> ((hi.lo)=w325:u64)
            n219 = Join Numbers(hi=w333, lo=w335) -> ((hi.lo)=w342:u64)
            n220 = Join Numbers(hi=fpga_settings."Feedback AM" ("FPGA Setting"), lo=w337) -> ((hi.lo)=w338:u64)
            n221 = Build Array(w338, w326, w325, w342) -> (w341:u64[])
            n222 = xnode "Invoke Method"("FPGA VI Reference In"=w343, "Data"=w341) -> ("FPGA VI Reference Out"=w322:T16)  [unwired: 2 in, 2 out]
            n223 = Bundle By Name(cluster=w345, "FPGA ref"=w322) -> (w344:T17)
          }
          event "ch0 DC offset": Value Change {
            n224 = event-data() -> ()  [unwired: 1 in, 6 out]
            n225 = Unbundle By Name(w359) -> ("FPGA ref"=w347:T16)
            n226 = Divide(x=32768, y=5) -> (x/y=w356:dbl)
            n227 = Multiply(x="ch0 DC offset", y=w356) -> (x*y=w355:dbl)
            n228 = Round To Nearest(number=w355) -> (nearest integer value=w354:dbl)
            n229 = To Word Integer(number=w354) -> (16bit integer=w348:i16)
            n230 = xnode "Reinterpret Number"("x"=w348) -> ("y"=w351:fxp<+/-,16,14>)
            n231 = xnode "Reinterpret Number"("x"=w351) -> ("y"=w350:fxp<+,16,16>)
            n232 = call "Write 16bit value.vi"("value"=w350, "FPGA Setting"=fpga_settings."DC_offs 0", "FPGA ref"=w347) -> ("FPGA ref out"=w346:T16)  [unwired: 7 in, 1 out]
            n233 = Bundle By Name(cluster=w359, "FPGA ref"=w346) -> (w358:T17)
          }
          event "ch1 DC offset": Value Change {
            n234 = event-data() -> ()  [unwired: 1 in, 6 out]
            n235 = Unbundle By Name(w373) -> ("FPGA ref"=w361:T16)
            n236 = Divide(x=32768, y=5) -> (x/y=w370:dbl)
            n237 = Multiply(x="ch1 DC offset", y=w370) -> (x*y=w369:dbl)
            n238 = Round To Nearest(number=w369) -> (nearest integer value=w368:dbl)
            n239 = To Word Integer(number=w368) -> (16bit integer=w362:i16)
            n240 = xnode "Reinterpret Number"("x"=w362) -> ("y"=w365:fxp<+/-,16,14>)
            n241 = xnode "Reinterpret Number"("x"=w365) -> ("y"=w364:fxp<+,16,16>)
            n242 = call "Write 16bit value.vi"("value"=w364, "FPGA Setting"=fpga_settings."DC_offs 1", "FPGA ref"=w361) -> ("FPGA ref out"=w360:T16)  [unwired: 7 in, 1 out]
            n243 = Bundle By Name(cluster=w373, "FPGA ref"=w360) -> (w372:T17)
          }
          event Value Change {
            n244 = event-data() -> ()  [unwired: 1 in, 6 out]
            n245 = Unbundle By Name(w377) -> ("FPGA ref"=w379:T16)
            n246 = property on="Rumode" class="Bool (strict)"("Val(Sgnl)"=FALSE ("Value (Signaling)")) -> ()  [unwired: 2 in, 2 out]
            n247 = xnode "Read/Write Control"("FPGA VI Reference In"=w379, "Mode"="Mode") -> ("FPGA VI Reference Out"=w378:T16)  [unwired: 1 in, 1 out]
            n248 = Bundle By Name(cluster=w377, "FPGA ref"=w378, "data mode"="Mode") -> (w376:T17)
          }
          event Value Change {
            n249 = event-data() -> ()  [unwired: 1 in, 6 out]
            n250 = Bundle By Name(cluster=w381, "5782 Trigger"="Trigger") -> (w380:T17)
          }
          event "Samples per 5782 record": Value Change {
            n251 = event-data() -> ()  [unwired: 1 in, 6 out]
            n252 = Unbundle By Name(w384) -> ("FPGA ref"=w387:T16)
            n253 = xnode "Read/Write Control"("FPGA VI Reference In"=w387, "5782 record length"="Samples per 5782 record") -> ("FPGA VI Reference Out"=w386:T16)  [unwired: 1 in, 1 out]
            n254 = Bundle By Name(cluster=w384, "FPGA ref"=w386, "samples per record"="Samples per 5782 record") -> (w383:T17)
          }
          event "Singleshot": Value Change {
            n255 = event-data() -> ()  [unwired: 1 in, 6 out]
            n256 = local write "Rumode"(FALSE ("Rumode")) -> ()
            n257 = Bundle By Name(cluster=w394, "scope mode"=ScopeMode."Single") -> (w389:T17)
            n258 = call "ToggleContinousMode.vi"("Cont Acquisition"=FALSE, "scope in"=w389) -> ("scope out"=w388:T17)  [unwired: 8 in, 1 out]
            n259 = call "ToggleAqcuisitionRunning_5782.vi"("Acquisition running"=TRUE, "scope in"=w388) -> ("scope out"=w392:T17)  [unwired: 8 in, 1 out]
            n260 = call "SendSWtrigger_5782.vi"("scope in"=w392) -> ("scope out"=w391:T17)  [unwired: 9 in, 1 out]
          }
          event "Rumode": Value Change {
            n261 = event-data() -> ()  [unwired: 1 in, 6 out]
            n262 = case shown="\"Triggered\"" "Trigmode" {
              tunnel: [ScopeMode."Running" ("scope mode") ScopeMode."Continuous" ("scope mode")] -> w397
              frame "Triggered" {
              }
              frame "Continuous" {
              }
            }
            n263 = Select(t=w397, s="Rumode", f=ScopeMode."Stopped" ("scope mode")) -> (s? t:f=w401:T18)
            n264 = Bundle By Name(cluster=w402, "scope mode"=w401) -> (w400:T17)
            n265 = case shown="\"Single\", \"Running\"" w401 {
              tunnel: w400 -> [w409 w416 w420]
              tunnel: [w410 w414 w421] -> w399
              frame "Single", "Running" {
                n266 = call "ToggleContinousMode.vi"("Cont Acquisition"=FALSE, "scope in"=w409) -> ("scope out"=w407:T17)  [unwired: 8 in, 1 out]
                n267 = call "ToggleAqcuisitionRunning_5782.vi"("Acquisition running"=TRUE, "scope in"=w407) -> ("scope out"=w411:T17)  [unwired: 8 in, 1 out]
                n268 = call "SendSWtrigger_5782.vi"("scope in"=w411) -> ("scope out"=w410:T17)  [unwired: 9 in, 1 out]
              }
              frame "Continuous" {
                n269 = call "ToggleAqcuisitionRunning_5782.vi"("Acquisition running"=TRUE, "scope in"=w416) -> ("scope out"=w415:T17)  [unwired: 8 in, 1 out]
                n270 = call "ToggleContinousMode.vi"("Cont Acquisition"=TRUE ("Acquisition running"), "scope in"=w415) -> ("scope out"=w414:T17)  [unwired: 8 in, 1 out]
              }
              frame "Stopped" {
                n271 = call "ToggleContinousMode.vi"("Cont Acquisition"=FALSE, "scope in"=w420) -> ("scope out"=w418:T17)  [unwired: 8 in, 1 out]
                n272 = call "ToggleAqcuisitionRunning_5782.vi"("Acquisition running"=FALSE, "scope in"=w418) -> ("scope out"=w421:T17)  [unwired: 8 in, 1 out]
              }
            }
          }
          event Value Change {
            n273 = event-data() -> ("CtlRef"=w425:refnum<vi>, "NewVal"=w423:bool)  [unwired: 1 in, 4 out]
            n274 = Search 1D Array(1D array=w426, element=w425) -> (index of element=w424:i32)  [unwired: 1 in]
            n275 = property on="Upper graph" class="WFGraph (strict)"("Active Plot"=w424, "Plot.Visible?"=w423) -> ()  [unwired: 2 in, 2 out]
            n276 = property on="Upper chart" class="WFChart (strict)"("Active Plot"=w424, "Plot.Visible?"=w423) -> ()  [unwired: 2 in, 2 out]
          }
          event Value Change {
            n277 = event-data() -> ("CtlRef"=w437:refnum<vi>, "NewVal"=w429:bool)  [unwired: 1 in, 4 out]
            n278 = local read "unwrap phase"() -> (w431:bool)
            n279 = Search 1D Array(1D array=w436, element=w437) -> (index of element=w435:i32)  [unwired: 1 in]
            n280 = Add(x=w435, y=2) -> (x+y=w433:i32)
            n281 = property on="freqdata" class="WFGraph (strict)"("Active Plot"=w435, "Plot.Visible?"=w429) -> ()  [unwired: 2 in, 2 out]
            n282 = Not(x=w431) -> (.not. x?=w430:bool)
            n283 = And(x=w431, y=w429) -> (x .and. y?=w432:bool)
            n284 = And(x=w430, y=w429) -> (x .and. y?=w428:bool)
            n285 = property on="Lower chart" class="WFChart (strict)"("Active Plot"=w435, "Plot.Visible?"=w428, "Active Plot"=w433, "Plot.Visible?"=w432) -> ()  [unwired: 2 in, 2 out]
          }
          event "unwrap phase": Value Change {
            n286 = event-data() -> ()  [unwired: 1 in, 6 out]
            n287 = local read "Ch0"() -> (w441:bool)
            n288 = local read "Ch1"() -> (w443:bool)
            n289 = Not(x="unwrap phase") -> (.not. x?=w446:bool)
            n290 = And(x=w441, y=w446) -> (x .and. y?=w445:bool)
            n291 = And(x=w443, y=w446) -> (x .and. y?=w444:bool)
            n292 = And(x=w443, y="unwrap phase") -> (x .and. y?=w442:bool)
            n293 = And(x=w441, y="unwrap phase") -> (x .and. y?=w439:bool)
            n294 = property on="Lower chart" class="WFChart (strict)"("Active Plot"=u32 0, "Plot.Visible?"=w445, "Active Plot"=u32 1, "Plot.Visible?"=w444) -> ()  [unwired: 2 in, 2 out]
            n295 = property on="Lower chart" class="WFChart (strict)"("Active Plot"=u32 2, "Plot.Visible?"=w442, "Active Plot"=u32 3, "Plot.Visible?"=w439) -> ()  [unwired: 2 in, 2 out]
          }
          event User Event {
            n296 = event-data() -> ("Sender"=w454:string, "Variant"=w453:variant, "driver status"=w452:T13)  [unwired: 1 in, 5 out]
            n297 = Unbundle By Name(w456) -> ("RemoteConnection"=w458:refnum<class "RemoteConnection.lvclass">)
            n298 = call "HandleRemoteMessage.vi"("driver status"=w452, "Message data"=w453, "Sender"=w454, "RemoteConnection in"=w458) -> ("RemoteConnection out"=w457:refnum<class "RemoteConnection.lvclass">)  [unwired: 6 in, 1 out]
            n299 = Bundle By Name(cluster=w456, "RemoteConnection"=w457) -> (w455:T17)
          }
          event "stop": Value Change {
            n300 = event-data() -> ()  [unwired: 1 in, 6 out]
          }
          event Value Change {
            n301 = event-data() -> ()  [unwired: 1 in, 6 out]
            n302 = case shown="\"V\"" "Unit" {
              tunnel: ["V" "dBV" "V^2"] -> w463
              frame "V" {
              }
              frame "dBV" {
              }
              frame "V^2" {
              }
            }
            n303 = Concatenate Strings("Amplitude [", w463, "]") -> (w461:string)
            n304 = property on="freqdata" class="WFGraph (strict)"("YScale.NameLbl.Text"=w461) -> ()  [unwired: 2 in, 2 out]
          }
          event "#bins": Value Change {
            n305 = event-data() -> ()  [unwired: 1 in, 6 out]
            n306 = local read "Upper chart"() -> (w472:dbl[][])
            n307 = local read "Window"() -> (w473:T8)
            n308 = local read "Unit"() -> (w474:T7)
            n309 = call "calc FFT.vi"("#bins"="#bins", "dt"=1e-06, "Unit"=w474, "Window"=w473, "data"=w472) -> ("Power Spectrum / PSD"=w471:cluster{"f0":dbl, "df":dbl, "magnitude":dbl[]}[])  [unwired: 6 in]
            n310 = local write "freqdata"(w471) -> ()
          }
          event "Zoom time X", "Zoom time Y": Value Change {
            n311 = event-data() -> ()  [unwired: 1 in, 6 out]
            n312 = control-ref of="Upper chart"() -> (w479:refnum<vi>)
            n313 = control-ref of="Upper graph"() -> (w480:refnum<vi>)
            n314 = call "setZoomTool.vi"("Zoom Y"="Zoom time Y", "Zoom  X"="Zoom time X", "reference"=w479) -> ()  [unwired: 9 in]
            n315 = call "setZoomTool.vi"("Zoom Y"="Zoom time Y", "Zoom  X"="Zoom time X", "reference"=w480) -> ()  [unwired: 9 in]
          }
          event "Zoom freq Y", "Zoom freq X": Value Change {
            n316 = event-data() -> ()  [unwired: 1 in, 6 out]
            n317 = control-ref of="Lower chart"() -> (w485:refnum<vi>)
            n318 = control-ref of="Lower graph"() -> (w484:refnum<vi>)
            n319 = control-ref of="freqdata"() -> (w486:refnum<vi>)
            n320 = call "setZoomTool.vi"("Zoom Y"="Zoom freq Y", "Zoom  X"="Zoom freq X", "reference"=w486) -> ()  [unwired: 9 in]
            n321 = call "setZoomTool.vi"("Zoom Y"="Zoom freq Y", "Zoom  X"="Zoom freq X", "reference"=w485) -> ()  [unwired: 9 in]
            n322 = call "setZoomTool.vi"("Zoom Y"="Zoom freq Y", "Zoom  X"="Zoom freq X", "reference"=w484) -> ()  [unwired: 9 in]
          }
          event Value Change {
            w490 = dbl[][] [] ("History Data")
            n323 = event-data() -> ()  [unwired: 1 in, 6 out]
            n324 = property on="Upper chart" class="WFChart (strict)"("History Data"=w490) -> ()  [unwired: 2 in, 2 out]
            n325 = property on="Lower chart" class="WFChart (strict)"("History Data"=w490) -> ()  [unwired: 2 in, 2 out]
            n326 = local write "freqdata"(cluster{"f0":dbl, "df":dbl, "magnitude":dbl[]}[] [] ("freqdata")) -> ()
            n327 = call "UpdateGraphs.vi"("Buffer mode"="Buffer", "Display mode"="Display", "Graph_refs"=w491) -> ()  [unwired: 9 in]
            n328 = property on="Zoom time X" class="Bool (strict)"("Val(Sgnl)"=TRUE ("Value (Signaling)")) -> ()  [unwired: 2 in, 2 out]
          }
        }
      }
      "stop 2" <- w118
    }
    frame Error {
    }
  }
  n329 = Unregister For Events(event registration refnum=w74) -> ()  [unwired: 1 in, 1 out]
  n330 = Unbundle By Name(w55) -> ("FPGA ref"=w82:T16, "RemoteConnection"=w16:refnum<class "RemoteConnection.lvclass">)
  n331 = flat-sequence {
    tunnel: w82 -> [w499]
    tunnel: w16 -> [w498]
    frame #0 {
      n332 = call "Close.vi"("RemoteConnection in"=w498) -> ()  [unwired: 9 in, 2 out]
      n333 = xnode "Close FPGA VI Reference"("FPGA VI Reference In"=w499) -> ()  [unwired: 1 in, 1 out]
      n334 = global write "global_stop.vi" "Stop"(TRUE ("Stop")) -> ()
    }
  }
